vi "Main.vi"(10 "Database Manager in":refnum<class "Database Manager.lvclass">, 11 "Module Admin":refnum<class "Delacor_lib_QMH_Module Admin.lvclass">) -> ()   [LabVIEW 2021, in "Database Manager.lvlib"]
doc: "This template is based off of the Queued Message Handler design pattern and the Queued Message Handler project template that ships with LabVIEW.\n\nThe main difference is that the queue is private to this module and communication between modules is performed via Broadcast and Request events.\n\nRequest events are wrapped in public API methods and are handled in the Event Handling Loop (EHL) of this VI. Any module can register for Broadcast events sent by this module. The EHL generates messages based on user interface actions.\n\nThe Message Handling Loop (MHL) processes messages generated by the EHL, or by other messages. The messages are string values, so new messages can be added easily to the Message Cases case structure in the MHL. Each message cluster can also provide an optional value for Message Data, which is a variant that can be converted to whatever message-specific data is required.\n_____\nBased on DQMH Dev Tools: Project Template 7.1.2.1547."
uses:
  Database Manager.lvlib
  <vilib>/Delacor/Delacor QMH/Libraries/Module Admin_class/Delacor_lib_QMH_Module Admin.lvclass
  Database Manager/Database Manager.lvclass
  Module Data--cluster.ctl
  <vilib>/Delacor/Delacor QMH/Libraries/Message Queue_class/Delacor_lib_QMH_Message Queue.lvclass/Delacor_lib_QMH_Message Queue.ctl
  Stop Argument--cluster.ctl
  <vilib>/Delacor/Delacor QMH/Libraries/Module Admin_class/Delacor_lib_QMH_Module Admin.lvclass/Delacor_lib_QMH_Module Admin.ctl
  Show Config data Argument--cluster.ctl
  Show Config data (Reply Payload)--cluster.ctl
  <vilib>/Utility/miscctls.llb/LVPointTypeDef.ctl
  Database Manager/Database Manager.lvclass/Database Manager.ctl
  <vilib>/Delacor/Delacor QMH/Libraries/Message Queue_class/Delacor_lib_QMH_Enqueue Message (Single).vi
  <vilib>/Delacor/Delacor QMH/Libraries/Module Admin_class/Delacor_lib_QMH_Get External Launch.vi
  <vilib>/Delacor/Delacor QMH/Libraries/Message Queue_class/Delacor_lib_QMH_Message Queue.lvclass
panel:
  out "error out":errorcluster
  out "Status":string
  in  "Simulate MHL Error":bool
  in  "Simulate EHL Error":bool
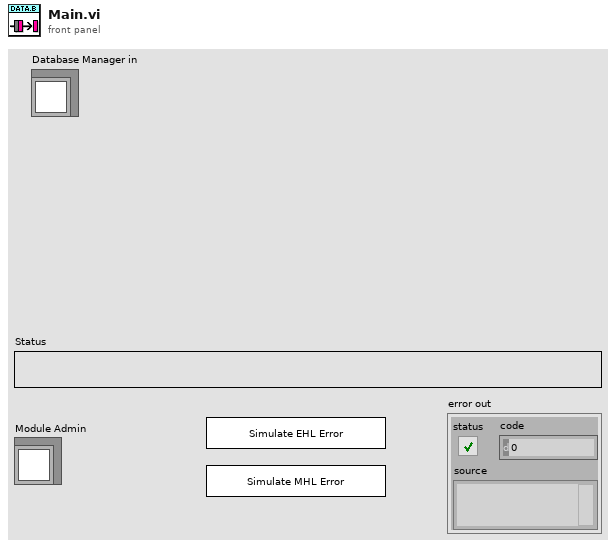
[diagram p1: front panel]
types:
  T1 = typedef "Database Manager.lvlib/Request Events--cluster.ctl" = cluster{"Stop Module":refnum<user-event>, "Show Panel":refnum<user-event>, "Hide Panel":refnum<user-event>, "Get Module Execution Status":refnum<user-event>, "Show Diagram":refnum<user-event>, "Show Config data":refnum<user-event>}
  T2 = typedef "Database Manager.lvlib/Module Data--cluster.ctl" = cluster{"Status":string}
  T3 = enum32{"invalid lock state", "Not Locked", "Locked (No Password)", "Password-protected"}
  T4 = typedef "Database Manager.lvlib/Stop Argument--cluster.ctl" = cluster{"Origin":string, "Exit via Stop Module Req?":bool, "Wait for Module to stop?":bool}
  T5 = typedef "Database Manager.lvlib/Show Config data Argument--cluster.ctl" = cluster{"Wait Notifier":refnum<notifier>, "wait for reply":bool}
  T6 = typedef "LVPointTypeDef.ctl" = cluster{"Horizontal":i16, "Vertical":i16}
  T7 = enum32{"Invalid", "Standard", "Closed", "Hidden", "Minimized", "Maximized"}
  T8 = cluster{"Path":path, "Params":cluster{"db_type":string, "host":string, "port":i32}}
  T9 = typedef "Database Manager.lvlib/Show Config data (Reply Payload)--cluster.ctl" = cluster{"Cluster of class private data":cluster{"Path":path, "Params":cluster{"db_type":string, "host":string, "port":i32}}, "error":errorcluster}
  T10 = cluster{"db_type":string, "host":string, "port":i32}
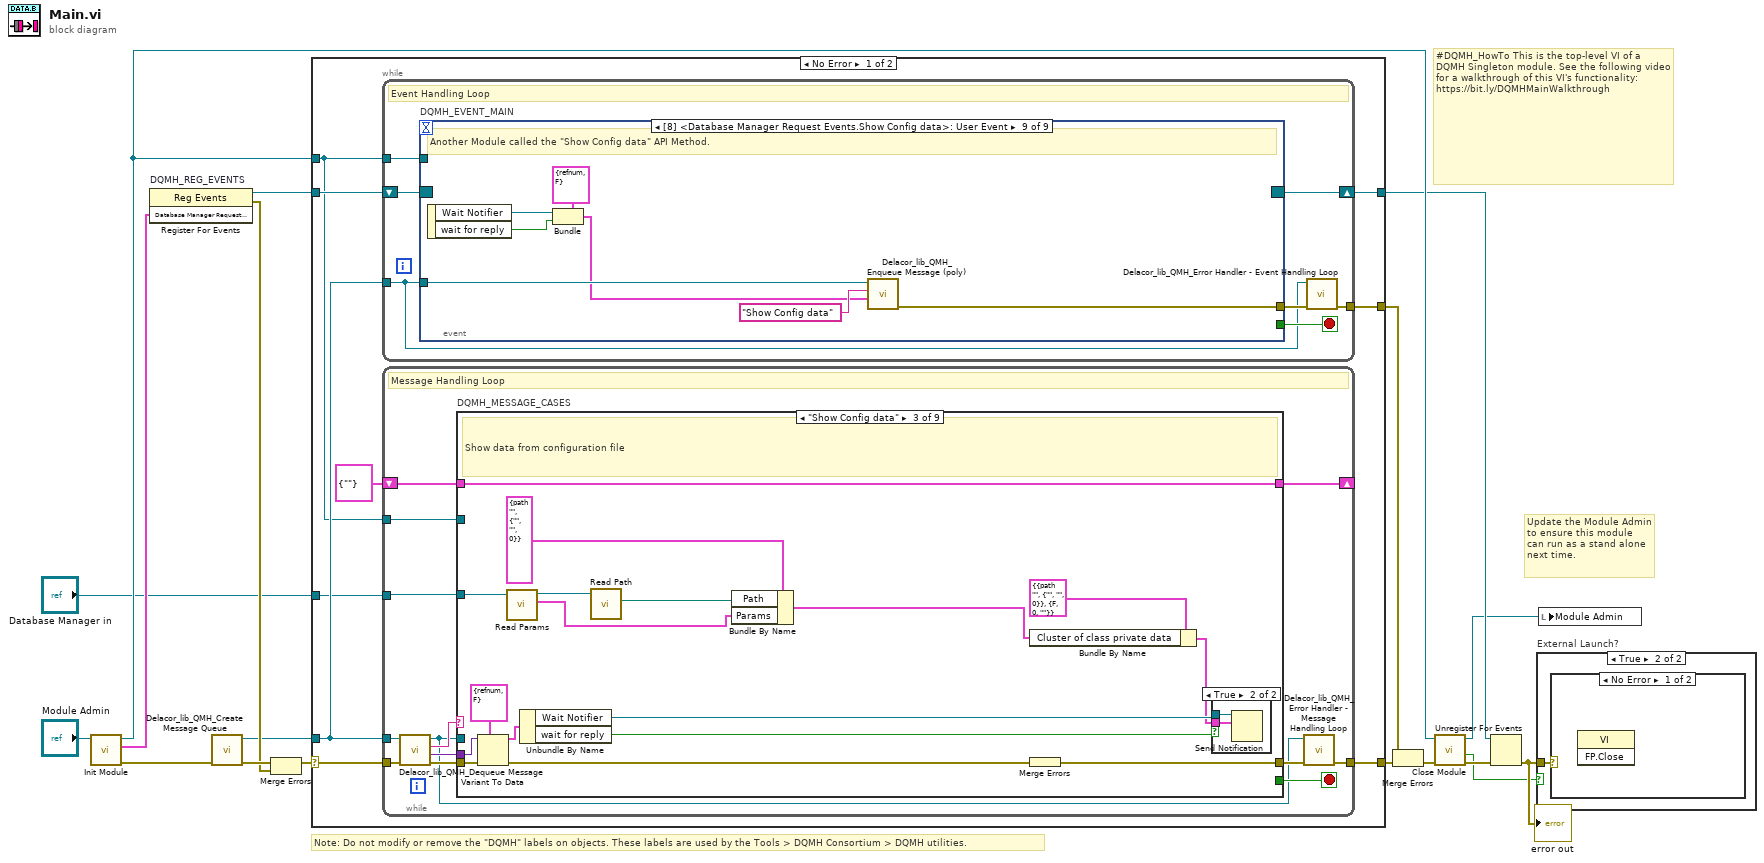
[diagram p0: block diagram]
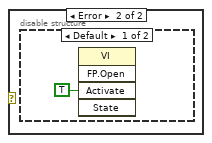
[diagram p3: hidden frame]
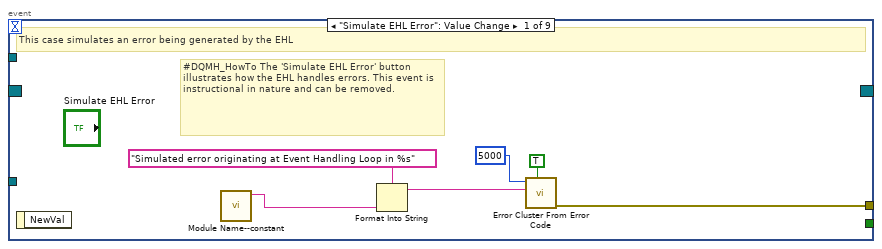
[diagram p5: hidden frame]
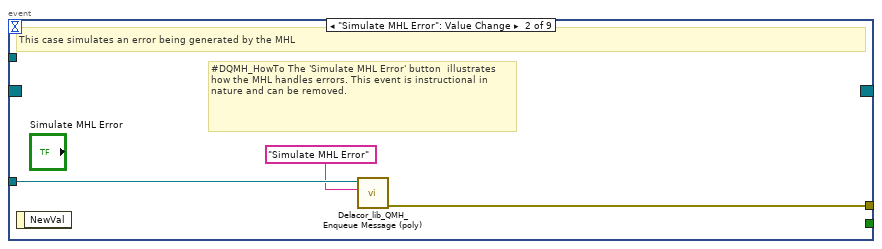
[diagram p6: hidden frame]
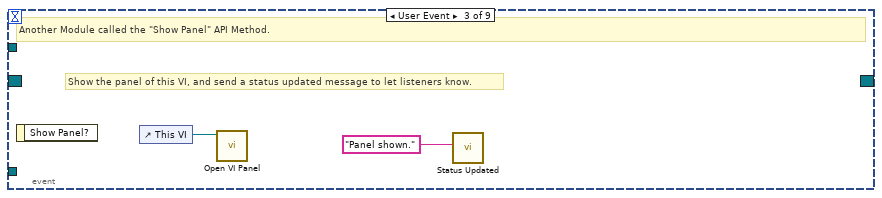
[diagram p7: hidden frame]
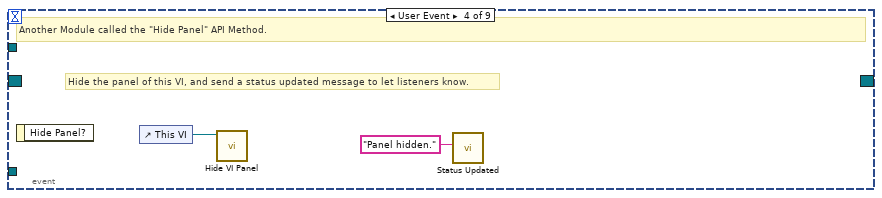
[diagram p8: hidden frame]
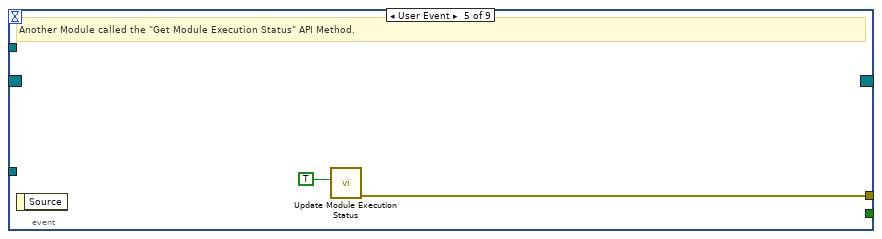
[diagram p9: hidden frame]
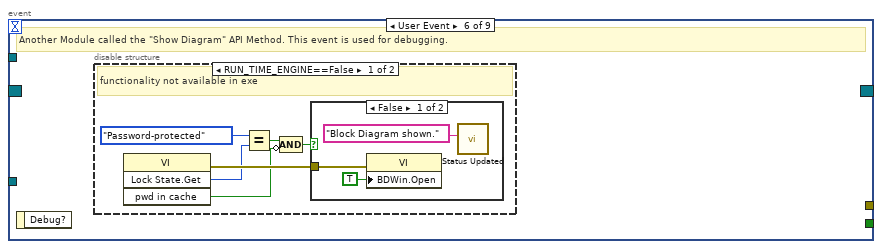
[diagram p10: hidden frame]
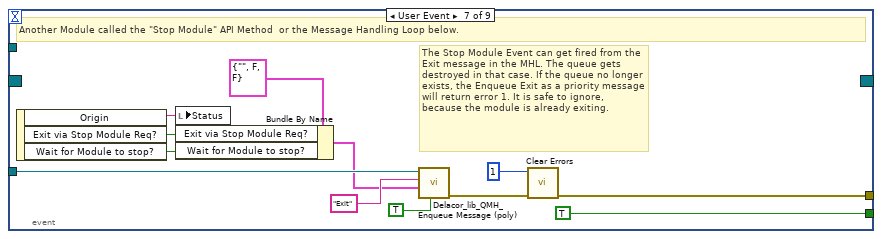
[diagram p13: hidden frame]
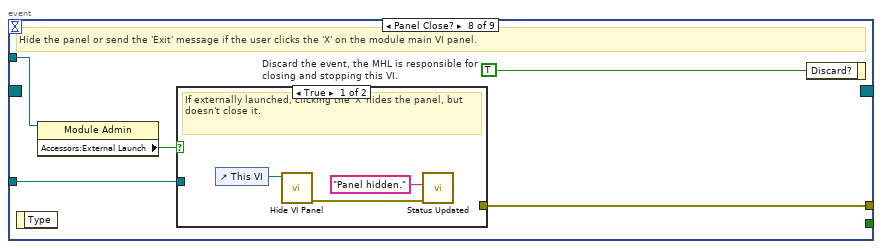
[diagram p14: hidden frame]
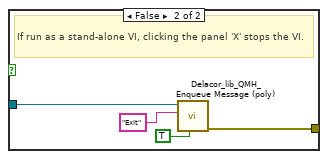
[diagram p15: hidden frame]
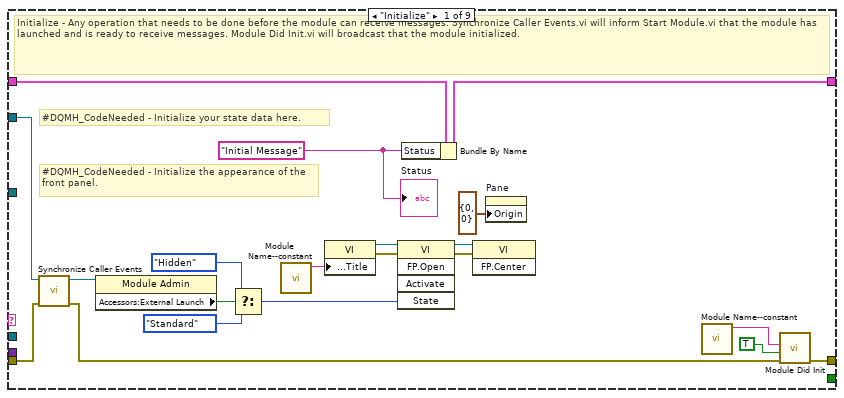
[diagram p16: hidden frame]
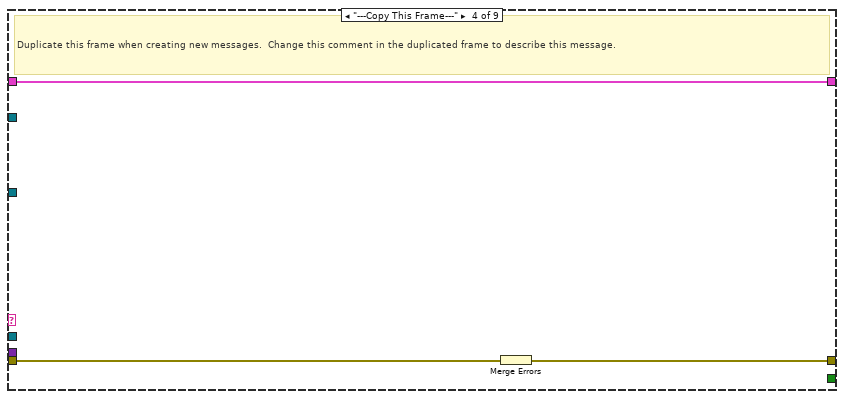
[diagram p19: hidden frame]
diagram:
  # "#DQMH_HowTo This is the top-level VI of a DQMH Singleton module. See the following video for a walkthrough of this VI's functionality: https://bit.ly/DQMHMainWalkthrough"
  # "Note: Do not modify or remove the \"DQMH\" labels on objects. These labels are used by the Tools > DQMH Consortium > DQMH utilities."
  # "Update the Module Admin to ensure this module can run as a stand alone next time."
  n1 = call "Init Module.vi"("Singleton Module Admin in"="Module Admin") -> ("error out"=w17:errorcluster, "Database Manager Request Events"=w6:T1, "Singleton Module Admin out"=w9:refnum<class "Delacor_lib_QMH_Module Admin.lvclass">)  [unwired: 8 in]
  n2 = register-events "DQMH_REG_EVENTS"(w6) -> (reference out=w7:refnum<event-registration>, error out=w10:errorcluster)  [unwired: 2 in]
  n3 = call <vilib>:"Delacor_lib_QMH_Create Message Queue.vi"("error in"=w17) -> ("error out"=w12:errorcluster, "Message Queue"=w5:refnum<class "Delacor_lib_QMH_Message Queue.lvclass">)  [unwired: 9 in]
  n4 = Merge Errors(w12, w10) -> (w11:errorcluster)
  n5 = case shown="No Error" w11 {
    selector: w11 -> [w25 w207]
    tunnel: [w27 w206] -> w18
    tunnel: [w24 w205] -> w8
    tunnel: w7 -> [w22 w205]
    tunnel: w5 -> [w21 w200]
    tunnel: [w26 _] -> w15
    tunnel: w9 -> [w20 w201]
    tunnel: "Database Manager in" -> [w19 _]
    frame No Error {
      n6 = while {
        tunnel: w21 -> [w28]
        shift-right: [w31] -> w24
        shift-left: w22 -> [w32]
        tunnel: [w33] -> w26
        tunnel: w20 -> [w29]
        stop <- w30 stop-if-true
        # "Event Handling Loop"
        n7 = event "DQMH_EVENT_MAIN" shown="[8] <Database Manager Request Events.Show Config data>: User Event" {
          selector: w32 -> [_ _ _ _ _ _ _ _ _]
          dyn-events: [_ _ _ _ _ _ _ _ _] -> w31
          timeout: _ -> [_ _ _ _ _ _ _ _ _]
          tunnel: [_ _ _ _ _ _ TRUE ("Discard?") _ _] -> w30
          tunnel: w28 -> [_ w42 _ _ _ _ w66 w73 w89]
          tunnel: [w40 w43 _ _ w49 _ w69 w75 w83] -> w34
          tunnel: w29 -> [_ _ _ _ _ _ _ w72 _]
          event "Simulate EHL Error": Value Change {
            # "#DQMH_HowTo The 'Simulate EHL Error' button  illustrates how the EHL handles errors. This event is instructional in nature and can be removed."
            # "This case simulates an error being generated by the EHL"
            n8 = event-data() -> ()  [unwired: 1 in, 1 out]
            n9 = call "Module Name--constant.vi"() -> ("Module Name"=w37:string)  [unwired: 11 in]
            n10 = Format Into String(format string="Simulated error originating at Event Handling Loop in %s", w37) -> (resulting string=w38:string)  [unwired: 2 in, 1 out]
            n11 = call <vilib>:"Error Cluster From Error Code.vi"("show call chain? (False)"=TRUE, "error message (\"\")"=w38, "error code (0)"=5000) -> ("error out"=w40:errorcluster)  [unwired: 6 in]
          }
          event "Simulate MHL Error": Value Change {
            # "#DQMH_HowTo The 'Simulate MHL Error' button  illustrates how the MHL handles errors. This event is instructional in nature and can be removed."
            # "This case simulates an error being generated by the MHL"
            n12 = event-data() -> ()  [unwired: 1 in, 1 out]
            n13 = call-poly <vilib>:"Delacor_lib_QMH_Enqueue Message (poly).vi"("Message"="Simulate MHL Error", "Message Queue in"=w42) -> ("error out"=w43:errorcluster)  [unwired: 8 in, 1 out]
          }
          event User Event {
            # "Show the panel of this VI, and send a status updated message to let listeners know."
            # "Another Module called the \"Show Panel\" API Method."
            n14 = event-data() -> ()  [unwired: 1 in, 1 out]
            n15 = control-ref of="This VI"() -> (w45:refnum<vi>)
            n16 = call "Open VI Panel.vi"("VI"=w45) -> ()  [unwired: 10 in, 1 out]
            n17 = call "Status Updated.vi"("Status"="Panel shown." ("format string")) -> ()  [unwired: 10 in, 1 out]
          }
          event User Event {
            # "Hide the panel of this VI, and send a status updated message to let listeners know."
            # "Another Module called the \"Hide Panel\" API Method."
            n18 = event-data() -> ()  [unwired: 1 in, 1 out]
            n19 = control-ref of="This VI"() -> (w47:refnum<vi>)
            n20 = call "Hide VI Panel.vi"("VI"=w47) -> ()  [unwired: 10 in, 1 out]
            n21 = call "Status Updated.vi"("Status"="Panel hidden." ("format string")) -> ()  [unwired: 10 in, 1 out]
          }
          event User Event {
            # "Another Module called the \"Get Module Execution Status\" API Method."
            n22 = event-data() -> ()  [unwired: 1 in, 1 out]
            n23 = call "Update Module Execution Status.vi"("Running?"=TRUE) -> ("error out"=w49:errorcluster)  [unwired: 10 in]
          }
          event User Event {
            # "Another Module called the \"Show Diagram\" API Method. This event is used for debugging."
            n24 = event-data() -> ()  [unwired: 1 in, 1 out]
            n25 = disable-structure shown="RUN_TIME_ENGINE==False" {
              frame condition #0 (active) {
                # "functionality not available in exe"
                n26 = invoke on="Invoke Node" class="VI" method="Lock State.Get"() -> (error out=w55:errorcluster, "Get Lock State"=w54:T3, "pwd in cache"=w51:bool)  [unwired: 4 in, 1 out]
                n27 = Equal?(x=T3."Password-protected", y=w54) -> (x = y?=w52:bool)
                n28 = Compound Arithmetic op=AND(w52, invert w51) -> (w50:bool)
                n29 = case shown="False" w50 {
                  tunnel: w55 -> [w58 _]
                  frame False {
                    n30 = property on="Property Node" class="VI"(error in=w58, "BDWin.Open"=TRUE ("Block Diagram Window:Open")) -> ()  [unwired: 1 in, 2 out]
                    n31 = call "Status Updated.vi"("Status"="Block Diagram shown." ("format string")) -> ()  [unwired: 10 in, 1 out]
                  }
                  frame True {
                    # "Password-protected VI, and the password is not in the cache. Do not show the diagram."
                  }
                }
              }
              frame condition #1 {
              }
            }
          }
          event User Event {
            # "The Stop Module Event can get fired from the Exit message in the MHL. The queue gets destroyed in that case. If the queue no longer exists, the Enqueue Exit as a priority message will return error 1. It is safe to ignore, because the module is already exiting."
            # "Another Module called the \"Stop Module\" API Method  or the Message Handling Loop below."
            n32 = event-data() -> ("Origin"=w65:string, "Exit via Stop Module Req?"=w61:bool, "Wait for Module to stop?"=w60:bool)  [unwired: 1 in]
            n33 = local write "Status"(w65) -> ()
            n34 = Bundle By Name(cluster=T4 {"Origin"="", "Exit via Stop Module Req?"=FALSE, "Wait for Module to stop?"=FALSE} ("Stop Argument"), "Exit via Stop Module Req?"=w61, "Wait for Module to stop?"=w60) -> (w59:T4)
            n35 = call-poly <vilib>:"Delacor_lib_QMH_Enqueue Message (poly).vi"("Priority Message? (F)"=TRUE, "Message Data"=w59, "Message"="Exit", "Message Queue in"=w66) -> ("error out"=w70:errorcluster)  [unwired: 6 in, 1 out]
            n36 = call <vilib>:"Clear Errors.vi"("error in (no error)"=w70, "specific error code to clear (0: all)"=1) -> ("error out"=w69:errorcluster)  [unwired: 4 in, 1 out]
          }
          event Panel Close? {
            w74 = TRUE  # Discard the event, the MHL is responsible for closing and stopping this VI.
            # "Hide the panel or send the 'Exit' message if the user clicks the 'X' on the module main VI panel."
            n37 = event-data() -> ()  [unwired: 1 in, 1 out]
            n38 = property on="Property Node" class="Module Admin"(reference=w72) -> ("Accessors:External Launch"=w71:bool)  [unwired: 1 in, 2 out]
            n39 = case shown="True" w71 {
              tunnel: w73 -> [_ w81]
              tunnel: [_ w82] -> w75
              frame True {
                # "If externally launched, clicking the 'X' hides the panel, but doesn't close it."
                n40 = control-ref of="This VI"() -> (w78:refnum<vi>)
                n41 = call "Hide VI Panel.vi"("VI"=w78) -> ("error out"=w76:errorcluster)  [unwired: 10 in]
                n42 = call "Status Updated.vi"("error in"=w76, "Status"="Panel hidden." ("format string")) -> ()  [unwired: 9 in, 1 out]
              }
              frame False {
                # "If run as a stand-alone VI, clicking the panel 'X' stops the VI."
                n43 = call-poly <vilib>:"Delacor_lib_QMH_Enqueue Message (poly).vi"("Priority Message? (F)"=TRUE, "Message"="Exit", "Message Queue in"=w81) -> ("error out"=w82:errorcluster)  [unwired: 7 in, 1 out]
              }
            }
            n44 = event-data ("Event Filter Node")("Discard?"=w74) -> ()  [unwired: 1 in, 1 out]
          }
          event User Event {
            # "Another Module called the \"Show Config data\" API Method."
            n45 = event-data() -> ("Wait Notifier"=w85:refnum<notifier>, "wait for reply"=w84:bool)  [unwired: 1 in]
            n46 = Bundle(cluster=T5 {"Wait Notifier"=refnum, "wait for reply"=FALSE} ("Show Config data Argument"), "Wait Notifier"=w85, "wait for reply"=w84) -> (w86:T5)
            n47 = call-poly <vilib>:"Delacor_lib_QMH_Enqueue Message (poly).vi"("Message Data"=w86, "Message"="Show Config data", "Message Queue in"=w89) -> ("error out"=w83:errorcluster)  [unwired: 7 in, 1 out]
          }
        }
        n48 = call-dynamic "Delacor_lib_QMH_Error Handler - Event Handling Loop.vi"("error in"=w34, "Message Queue in"=w28) -> ("dup error in"=w33:errorcluster)  [unwired: 8 in, 1 out]
      }
      n49 = while {
        tunnel: w21 -> [w91]
        shift-right: [w99] -> _
        shift-left: T2 {"Status"=""} ("Data Cluster") -> [w100]
        tunnel: w25 -> [w102]
        tunnel: [w94] -> w27
        tunnel: w20 -> [w95]
        tunnel: w19 -> [w90]
        stop <- w98 stop-if-true
        # "Message Handling Loop"
        n50 = call-dynamic "Delacor_lib_QMH_Dequeue Message.vi"("error in"=w102, "Message Queue in"=w91) -> ("error out"=w101:errorcluster, "Message Data"=w96:variant, "Message"=w97:string, "Message Queue out"=w92:refnum<class "Delacor_lib_QMH_Message Queue.lvclass">)  [unwired: 6 in]
        n51 = case "DQMH_MESSAGE_CASES" shown="\"Show Config data\"" w97 {
          selector: w97 -> [_ _ _ _ _ _ _ _ w195]
          tunnel: w92 -> [_ _ _ _ _ _ w161 w183 _]
          tunnel: w101 -> [w120 w124 w141 w146 w148 w157 w168 w189 w198]
          tunnel: [w118 w124 w131 w145 w148 w156 w164 w184 w199] -> w93
          tunnel: w100 -> [w109 w123 w140 w144 w147 w154 w163 w182 w196]
          tunnel: [w108 w123 w140 w144 w147 w154 w163 w182 w196] -> w99
          tunnel: [_ _ _ _ _ _ _ w181 _] -> w98
          tunnel: w96 -> [_ _ w138 _ _ _ w162 w180 _]
          tunnel: w95 -> [w110 _ _ _ _ _ w160 w175 _]
          tunnel: w90 -> [_ _ w130 _ _ _ _ _ _]
          frame "Initialize" {
            w104 = "Initial Message" ("Initial Message")
            # "#DQMH_CodeNeeded - Initialize the appearance of the front panel."
            # "#DQMH_CodeNeeded - Initialize your state data here."
            # "Initialize - Any operation that needs to be done before the module can receive messages. Synchronize Caller Events.vi will inform Start Module.vi that the module has launched and is ready to receive messages. Module Did Init.vi will broadcast that the module initialized."
            n52 = call "Synchronize Caller Events.vi"("error in"=w120, "Singleton Module Admin in"=w110) -> ("error out"=w119:errorcluster, "Singleton Module Admin out"=w105:refnum<class "Delacor_lib_QMH_Module Admin.lvclass">)  [unwired: 8 in]
            n53 = property on="Property Node" class="Module Admin"(reference=w105) -> ("Accessors:External Launch"=w114:bool)  [unwired: 1 in, 2 out]
            n54 = Select(t=T7."Hidden" ("State"), s=w114, f=T7."Standard" ("State")) -> (s? t:f=w111:T7)
            n55 = call "Module Name--constant.vi"() -> ("Module Name"=w117:string)  [unwired: 11 in]
            n56 = property on="Property Node" class="VI"("Front Panel.Title"=w117) -> (reference out=w116:refnum<vi>, error out=w122:errorcluster)  [unwired: 2 in]
            n57 = invoke on="Invoke Node" class="VI" method="FP.Open"(reference=w116, error in=w122, "State"=w111) -> (reference out=w115:refnum<vi>, error out=w121:errorcluster)  [unwired: 2 in, 3 out]
            n58 = Bundle By Name(cluster=w109, "Status"=w104) -> (w108:T2)
            n59 = invoke on="Invoke Node" class="VI" method="FP.Center"(reference=w115, error in=w121) -> ()  [unwired: 1 in, 3 out]
            n60 = property on="Pane" class="Pane"("Origin"=T6 {"Horizontal"=0, "Vertical"=0}) -> ()  [unwired: 2 in, 2 out]
            n61 = call "Module Name--constant.vi"() -> ("Module Name"=w106:string)  [unwired: 11 in]
            n62 = call "Module Did Init.vi"("error in"=w119, "Initialized?"=TRUE, "Origin"=w106) -> ("error out"=w118:errorcluster)  [unwired: 8 in]
            "Status" <- w104
          }
          frame "---Module Specific---" {
            # "Separator -- The following cases handle messages specific to this Module."
          }
          frame "Show Config data" {
            # "Show data from configuration file"
            n63 = Variant To Data(error in=w141, type=T5 {"Wait Notifier"=refnum, "wait for reply"=FALSE} ("Show Config data Argument"), Variant=w138) -> (data=w136:T5, error out=w139:errorcluster)
            n64 = call "Read Params.vi"("Database Manager in"=w130) -> ("Params"=w126:T10, "Database Manager out"=w129:refnum<class "Database Manager.lvclass">)  [unwired: 8 in, 1 out]
            n65 = Unbundle By Name(w136) -> ("Wait Notifier"=w135:refnum<notifier>, "wait for reply"=w134:bool)
            n66 = call "Read Path.vi"("Database Manager in"=w129) -> ("Path"=w127:path)  [unwired: 8 in, 2 out]
            n67 = Bundle By Name(cluster=T8 {"Path"=path "", "Params"={"db_type"="", "host"="", "port"=0}} ("Cluster of class private data"), "Path"=w127, "Params"=w126) -> (w125:T8)
            n68 = Bundle By Name(cluster=T9 {"Cluster of class private data"={"Path"=path "", "Params"={"db_type"="", "host"="", "port"=0}}, "error"={"status"=FALSE, "code"=0, "source"=""}} ("Show Config data (Reply Payload)"), "Cluster of class private data"=w125) -> (w133:T9)
            n69 = Merge Errors(w139) -> (w131:errorcluster)
            n70 = case "DQMH_FIRE_NOTIFIER" shown="True" w134 {
              tunnel: w135 -> [_ w143]
              tunnel: w133 -> [_ w142]
              frame False {
              }
              frame True {
                n71 = Send Notification(notification=w142, notifier=w143) -> ()  [unwired: 1 in, 2 out]
              }
            }
          }
          frame "---Copy This Frame---" {
            # "Duplicate this frame when creating new messages.  Change this comment in the duplicated frame to describe this message."
            n72 = Merge Errors(w146) -> (w145:errorcluster)
          }
          frame "---Exit and Error Handling---" {
            # "Separator - The following cases handle errors and exit messages."
          }
          frame "Simulate MHL Error" {
            # "#DQMH_HowTo The 'Simulate MHL Error' button  illustrates how the MHL handles errors. This event is instructional in nature and can be removed."
            # "Simulate an error occurring at the MHL"
            n73 = call "Module Name--constant.vi"() -> ("Module Name"=w150:string)  [unwired: 11 in]
            n74 = Format Into String(format string="Simulated error originating at Message Handling Loop in %s", w150) -> (resulting string=w151:string)  [unwired: 2 in, 1 out]
            n75 = call <vilib>:"Error Cluster From Error Code.vi"("show call chain? (False)"=TRUE, "error message (\"\")"=w151, "error code (0)"=5001) -> ("error out"=w155:errorcluster)  [unwired: 6 in]
            n76 = Merge Errors(w157, w155) -> (w156:errorcluster)
          }
          frame "Error" {
            # "#DQMH_CodeRecommended - If the module is running in standalone mode (External Launch = FALSE), this code will pop up an error dialog and call the 'Exit' message if an error occurs. Add more fine-grained error management here."
            # "Error - Check the error message data and respond accordingly. This message is sent by the \"Error Handler\" VIs at the end of each loop in this application."
            n77 = property on="Property Node" class="Module Admin"(reference=w160) -> ("Accessors:External Launch"=w159:bool)  [unwired: 1 in, 2 out]
            n78 = Variant To Data(error in=w168, type=errorcluster {"status"=FALSE, "code"=0, "source"=""} ("error constant"), Variant=w162) -> (data=w158:errorcluster, error out=w166:errorcluster)
            n79 = local write "error out"(w158) -> ()
            n80 = call "Error Reported.vi"("Error"=w158) -> ()  [unwired: 10 in, 1 out]
            n81 = case shown="False" w159 {
              tunnel: [w173 _] -> w165
              tunnel: w161 -> [w171 _]
              tunnel: w158 -> [w172 _]
              frame False {
                n82 = disable-structure shown="Default" {
                  disable-tunnel: w172 -> [w174 _]
                  frame condition #0 (active) {
                    # "If the module is running standalone, then pop up an error dialog and call the \"Exit\" message."
                    n83 = call <vilib>:"Simple Error Handler.vi"("error in (no error)"=w174) -> ()  [unwired: 4 in, 5 out]
                  }
                  frame condition #1 {
                    # "To prevent the Simple Error Handler VI from being loaded (e.g. when deploying to a Real-Time target), add the Conditional Disable Symbol \"DQMH_Disable_SEH\" to your project and set it to TRUE."
                  }
                }
                n84 = call-poly <vilib>:"Delacor_lib_QMH_Enqueue Message (poly).vi"("Priority Message? (F)"=TRUE, "Message"="Exit", "Message Queue in"=w171) -> ("error out"=w173:errorcluster)  [unwired: 7 in, 1 out]
              }
              frame True {
                # "If the module was launched externally, calling the Error Reported broadcast VI is the only action performed by the \"Error\" message. The module's caller can then process the error appropriately."
              }
            }
            n85 = Merge Errors(w166, w165) -> (w164:errorcluster)
          }
          frame "Exit" {
            w179 = 91  # 91: not all Exit messages will have an argument
            w181 = TRUE  # Stop the VI
            # "Release the message queue reference"
            # "#DQMH_CodeNeeded - Add any required cleanup code here."
            # "Exit - Exit the application."
            n86 = Variant To Data(error in=w189, type=T4 {"Origin"="", "Exit via Stop Module Req?"=FALSE, "Wait for Module to stop?"=FALSE} ("Stop Argument"), Variant=w180) -> (data=w177:T4, error out=w186:errorcluster)
            n87 = call <vilib>:"Clear Errors.vi"("error in (no error)"=w186, "specific error code to clear (0: all)"=w179) -> ("error out"=w188:errorcluster)  [unwired: 4 in, 1 out]
            n88 = control-ref of="This VI"() -> (w176:refnum<vi>)
            n89 = call-dynamic "Delacor_lib_QMH_Release Message Queue.vi"("error in"=w188, "Message Queue"=w183) -> ("error out"=w187:errorcluster)  [unwired: 9 in]
            n90 = call "Handle Exit.vi"("Stop Argument"=w177, "Admin in"=w175, "VI reference"=w176) -> ("error out"=w185:errorcluster)  [unwired: 7 in, 1 out]
            n91 = Merge Errors(w187, w185) -> (w184:errorcluster)
            n92 = call "Error Reported.vi"("Error"=w184) -> ()  [unwired: 10 in, 1 out]
          }
          frame Default {
            # "'Default' case only runs if there is a message that isn't defined in any of the other cases.  Output a programming error."
            n93 = call "Module Name--constant.vi"() -> ("Module Name"=w194:string)  [unwired: 11 in]
            n94 = Format Into String(format string="The invalid message string \"%s\" was received in the Message Handling Loop for module \"%s\".", w195, w194) -> (resulting string=w190:string)  [unwired: 2 in, 1 out]
            n95 = call <vilib>:"Error Cluster From Error Code.vi"("show call chain? (False)"=TRUE, "error message (\"\")"=w190, "error code (0)"=1) -> ("error out"=w197:errorcluster)  [unwired: 6 in]
            n96 = Merge Errors(w198, w197) -> (w199:errorcluster)
          }
        }
        n97 = call-dynamic "Delacor_lib_QMH_Error Handler - Message Handling Loop.vi"("error in"=w93, "Message Queue in"=w92) -> ("dup error in"=w94:errorcluster)  [unwired: 8 in, 1 out]
      }
    }
    frame Error {
      # "Synchronize Caller Events.vi will inform Start Module.vi that the module has launched and will let the code calling Start Module.vi register for broadcasts and would permit the caller receive the broadcast that an error occurred at launch time."
      n98 = call-dynamic "Delacor_lib_QMH_Release Message Queue.vi"("error in"=w207, "Message Queue"=w200) -> ("error out"=w206:errorcluster)  [unwired: 9 in]
      n99 = call "Synchronize Caller Events.vi"("Singleton Module Admin in"=w201) -> ("error out"=w208:errorcluster)  [unwired: 9 in, 1 out]
      n100 = call "Module Name--constant.vi"() -> ("Module Name"=w204:string)  [unwired: 11 in]
      n101 = Format Into String(format string="An error occurred during initialization. %s is no longer running.", w204) -> (resulting string=w202:string)  [unwired: 2 in, 1 out]
      n102 = Merge Errors(w206, w208) -> (w209:errorcluster)
      n103 = call "Error Reported.vi"("Additional Information"=w202, "Error"=w209) -> ()  [unwired: 9 in, 1 out]
    }
  }
  n104 = Merge Errors(w15, w18) -> (w14:errorcluster)
  n105 = call "Close Module.vi"("error in"=w14, "Module Admin in"=w9) -> ("error out"=w16:errorcluster, "External Launch"=w2:bool, "Module Admin out"=w3:refnum<class "Delacor_lib_QMH_Module Admin.lvclass">)  [unwired: 7 in]
  n106 = Unregister For Events(event registration refnum=w8, error in=w16) -> (error out=w13:errorcluster)
  "error out" <- w13
  n107 = case "External Launch?" shown="True" w2 {
    tunnel: w13 -> [_ w210]
    frame False {
    }
    frame True {
      n108 = case shown="No Error" w210 {
        frame No Error {
          n109 = invoke on="Invoke Node" class="VI" method="FP.Close"() -> ()  [unwired: 3 in, 3 out]
        }
        frame Error {
          n110 = disable-structure shown="Default" {
            frame condition #0 (active) {
              n111 = invoke class="VI" method="FP.Open"("Activate"=TRUE ("Activate?")) -> ()  [unwired: 4 in, 5 out]
            }
            frame condition #1 {
              # "Don't show panel on error if running inside a built EXE."
            }
          }
        }
      }
    }
  }
  n112 = local write "Module Admin"(w3) -> ()
